vi "Create MetaData Channel - Single Channel - Type Cast.vi"(8 "error in (no error)":errorcluster, 9 "settings":T1, 10 "channel name":string, 11 "command refnum in":T4=18446744073709551615 format="%.0x") -> (0 "error out":errorcluster, 2 "channel refnum":T4=18446744073709551615 format="%.0x", 3 "command refnum out":T4=18446744073709551615 format="%.0x")   [LabVIEW 2018, in "Instrument Addon Scripting API.lvlib"]
doc: "Creates a new MetaData Channel under the specified command."
uses:
  Instrument Addon Scripting API.lvlib
  <vilib>/NI Veristand/Custom Device API/Custom Device Item Ref.ctl
  TypeDefs/Single Channel Type Cast Settings.ctl
  Addon/Addon Shared/Types/Type Cast Type.ctl
  Addon/Addon Shared/Types/Endian.ctl
  Addon/Addon Shared/Types/MetaData Parameters.ctl
  Addon/Addon Shared/Types/Protocol Data Type.ctl
  Addon/Addon Shared/Types/Metadata Channel Type.ctl
  TypeDefs/Channel Properties.ctl
  Addon/Addon Shared/Instrument Addon Shared.lvlib
  <vilib>/NI Veristand/Custom Device API/Custom Device API.lvlib
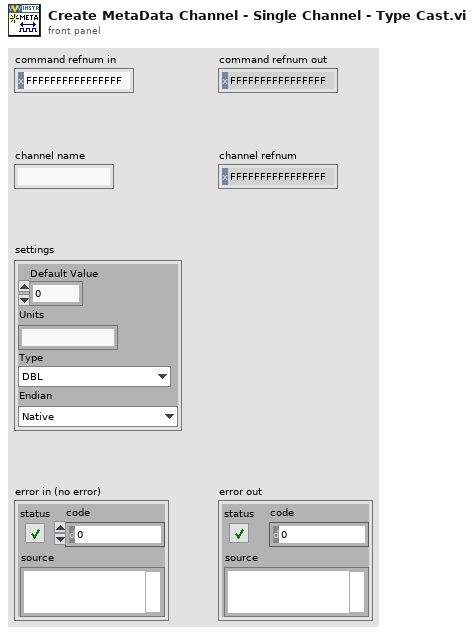
[diagram p1: front panel]
types:
  T1 = typedef "Instrument Addon Scripting API.lvlib/Single Channel Type Cast Settings.ctl" = cluster{"Default Value":dbl, "Units":string, "Type":T2, "Endian":T3}
  T2 = typedef "Instrument Addon Shared.lvlib/Type Cast Type.ctl" = enum16{"DBL", "SGL", "U64", "U32", "U16", "U8", "I64", "I32", "I16", "I8"}
  T3 = typedef "Instrument Addon Shared.lvlib/Endian.ctl" = enum16{"Native", "Little", "Big"}
  T4 = typedef "Custom Device API.lvlib/Custom Device Item Ref.ctl" = u64
  T5 = typedef "Instrument Addon Scripting API.lvlib/Channel Properties.ctl" = cluster{"Default Value":dbl, "Units":string}
  T6 = typedef "Instrument Addon Shared.lvlib/Metadata Channel Type.ctl" = enum16{"Enumerated List", "Format", "Type Cast"}
  T7 = typedef "Instrument Addon Shared.lvlib/Protocol Data Type.ctl" = enum16{"Single Channel", "Array"}
  T8 = typedef "Instrument Addon Shared.lvlib/MetaData Parameters.ctl" = cluster{"Data Type":T7, "Channel Type":T6, "List":string[], "Format String":string, "Type":T2, "Delimiter":string, "Endian":T3}
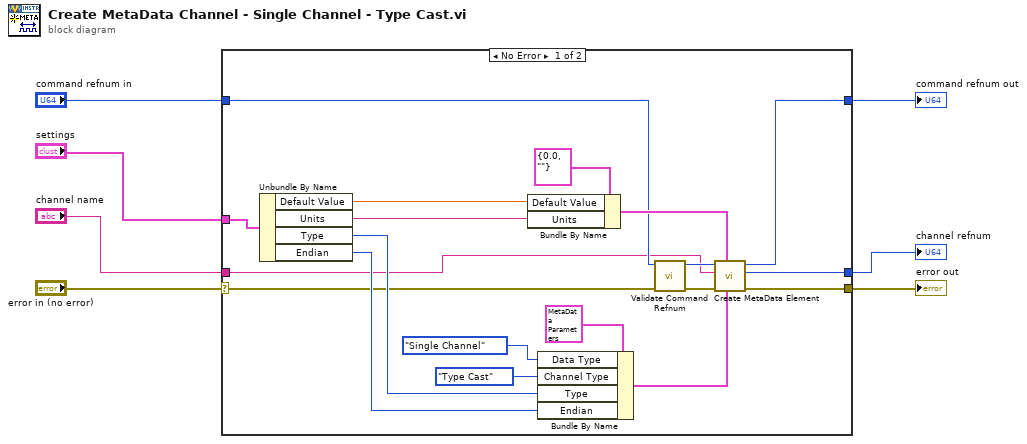
[diagram p0: block diagram]
diagram:
  n1 = case shown="No Error" "error in (no error)" {
    selector: "error in (no error)" -> [w11 w27]
    tunnel: [w26 w27] -> w7
    tunnel: "settings" -> [w25 _]
    tunnel: "command refnum in" -> [w10 w28]
    tunnel: [w15 _] -> w5
    tunnel: [w14 w28] -> w4
    tunnel: "channel name" -> [w8 _]
    frame No Error {
      n2 = Unbundle By Name(w25) -> ("Default Value"=w19:dbl, "Units"=w18:string, "Type"=w21:T2, "Endian"=w13:T3)
      n3 = Bundle By Name(cluster=T5 {"Default Value"=0.0, "Units"=""}, "Default Value"=w19, "Units"=w18) -> (w16:T5)
      n4 = Bundle By Name(cluster=T8 {"Data Type"=enum."Single Channel", "Channel Type"=enum."Format", "List"=[], "Format String"="%.3g", "Type"=enum."SGL", "Delimiter"="", "Endian"=enum."Native"} ("MetaData Parameters"), "Data Type"=Protocol_Data_Type."Single Channel", "Channel Type"=Metadata_Channel_Type."Type Cast", "Type"=w21, "Endian"=w13) -> (w20:T8)
      n5 = call "Validate Command Refnum.vi"("error in (no error)"=w11, "command refnum in"=w10) -> ("error out"=w12:errorcluster, "command refnum out"=w9:T4)  [unwired: 8 in]
      n6 = call "Create MetaData Element.vi"("MetaData Parameters"=w20, "Channel Properties"=w16, "error in (no error)"=w12, "Name"=w8, "Refnum In"=w9) -> ("error out"=w26:errorcluster, "Channel Refnum"=w15:T4, "Refnum Out"=w14:T4)  [unwired: 4 in]
    }
    frame Error {
    }
  }
  "command refnum out" <- w4
  "error out" <- w7
  "channel refnum" <- w5
